vi "9401_Update Lines.vi"(8 "error in":errorcluster, 9 "DIO7:4":u32(ring) items=["Input", "Output"], 10 "DIO3:0":u32(ring) items=["Input", "Output"], 11 "Node Ptr in":T1 format="%.0x") -> (0 "error out":errorcluster, 3 "Node Ptr out":T1 format="%.0x")   [LabVIEW 2019, in "Modules.lvlib" / "9401.lvclass"]
uses:
  9401.lvclass
  <vilib>/NI VeriStand/Custom Device API/Custom Device Item Ref.ctl
  C:/Users/nitest/Desktop/Git 2019/niveristand-scan-engine-module-libraries/Source/RSI Module/RSI Module.lvclass
  <vilib>/NI VeriStand/Custom Device API/Custom Device Channel Type.ctl
  9401.lvclass/9401.ctl
  RSI Module/Channel GUIDs.vi
  RSI Module/RSI Module.lvclass
  <vilib>/NI VeriStand/Custom Device API/Custom Device API.lvlib
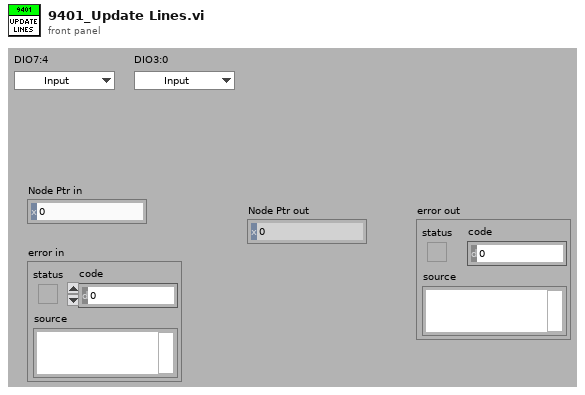
[diagram p1: front panel]
types:
  T1 = typedef "Custom Device API.lvlib/Custom Device Item Ref.ctl" = u64
  T2 = typedef "Custom Device API.lvlib/Custom Device Channel Type.ctl" = enum16{"Input", "Output"}
  T3 = typedef "Modules.lvlib/RSI Module.lvclass/Channels.ctl" = cluster{"# Input Channels":i32, "# Output Channels":i32, "Channel Type":T4, "Units":string}
  T4 = typedef "Modules.lvlib/RSI Module.lvclass/Channel Type.ctl" = enum16{"Analog", "Digital"}
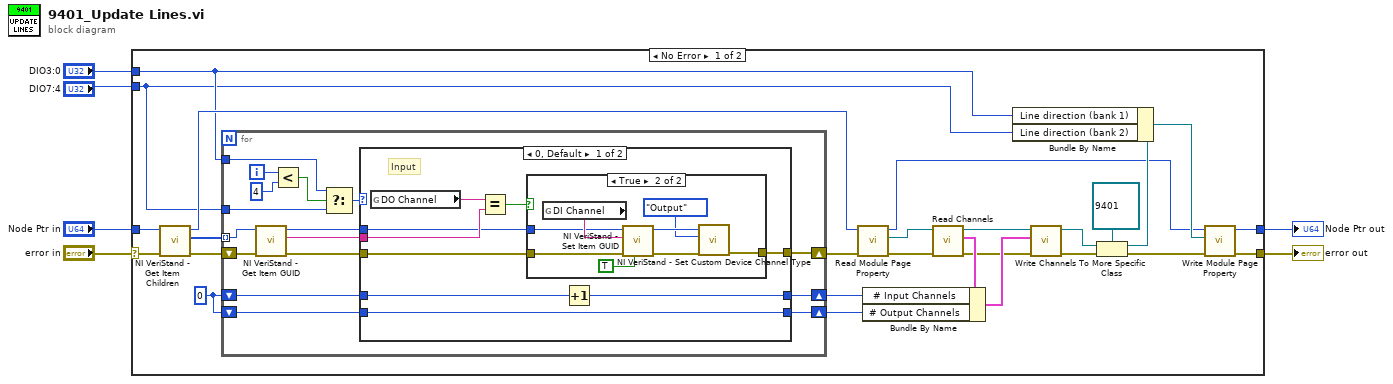
[diagram p0: block diagram]
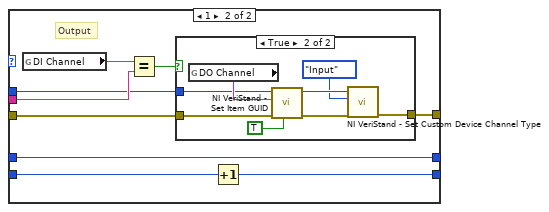
[diagram p3: hidden frame]
diagram:
  n1 = case shown="No Error" "error in" {
    selector: "error in" -> [w25 w86]
    tunnel: [w30 w86] -> w6
    tunnel: "Node Ptr in" -> [w24 w85]
    tunnel: [w26 w85] -> w4
    tunnel: "DIO3:0" -> [w20 _]
    tunnel: "DIO7:4" -> [w19 _]
    frame No Error {
      w18 = 0 ("# Input Channels")
      n2 = call <vilib>:"NI VeriStand - Get Item Children.vi"("error in (no error)"=w25, "Item Ref in"=w24) -> ("error out"=w22:errorcluster, "Child Refs"=w23:T1[], "Item Ref out"=w21:T1)  [unwired: 6 in, 1 out]
      n3 = for {
        tunnel: w23 -> [w47] mode=indexing
        shift-right: [w33] -> w17
        shift-left: w22 -> [w48]
        tunnel: w20 -> [w44]
        tunnel: w19 -> [w43]
        shift-right: [w35] -> w8
        shift-left: w18 -> [w37]
        shift-right: [w34] -> w7
        shift-left: w18 -> [w36]
        i -> [w46]
        n4 = call <vilib>:"NI VeriStand - Get Item GUID.vi"("error in (no error)"=w48, "Item Ref in"=w47) -> ("error out"=w38:errorcluster, "GUID"=w40:string, "Item Ref out"=w39:T1)  [unwired: 7 in]
        n5 = Less?(x=w46, y=4) -> (x < y?=w42:bool)
        n6 = Select(t=w44, s=w42, f=w43) -> (s? t:f=w41:u32)
        n7 = case shown="0, Default" w41 {
          tunnel: w40 -> [w56 w74]
          tunnel: w39 -> [w53 w71]
          tunnel: w38 -> [w54 w72]
          tunnel: [w52 w70] -> w33
          tunnel: w37 -> [w51 w67]
          tunnel: w36 -> [w49 w69]
          tunnel: [w50 w67] -> w35
          tunnel: [w49 w68] -> w34
          frame 0, Default {
            # "Input"
            n8 = global read "Channel GUIDs.vi" "DO Channel"() -> (w57:string)
            n9 = Equal?(x=w57, y=w56) -> (x = y?=w55:bool)
            n10 = case shown="True" w55 {
              tunnel: w54 -> [w58 w66]
              tunnel: w53 -> [_ w64]
              tunnel: [w58 w61] -> w52
              frame False {
              }
              frame True {
                n11 = global read "Channel GUIDs.vi" "DI Channel"() -> (w65:string)
                n12 = call <vilib>:"NI VeriStand - Set Item GUID.vi"("Refresh System Explorer Tree? (F)"=TRUE, "error in (no error)"=w66, "GUID"=w65, "Item Ref in"=w64) -> ("error out"=w62:errorcluster, "Item Ref out"=w63:T1)  [unwired: 6 in]
                n13 = call <vilib>:"NI VeriStand - Set Custom Device Channel Type.vi"("error in (no error)"=w62, "Type"=Custom_Device_Channel_Type."Output", "Channel Ref in"=w63) -> ("error out"=w61:errorcluster)  [unwired: 7 in, 1 out]
              }
            }
            n14 = Increment(x=w51) -> (x+1=w50:i32)
          }
          frame 1 {
            # "Output"
            n15 = global read "Channel GUIDs.vi" "DI Channel"() -> (w75:string)
            n16 = Equal?(x=w75, y=w74) -> (x = y?=w73:bool)
            n17 = case shown="True" w73 {
              tunnel: w72 -> [w76 w84]
              tunnel: w71 -> [_ w82]
              tunnel: [w76 w79] -> w70
              frame False {
              }
              frame True {
                n18 = global read "Channel GUIDs.vi" "DO Channel"() -> (w83:string)
                n19 = call <vilib>:"NI VeriStand - Set Item GUID.vi"("Refresh System Explorer Tree? (F)"=TRUE, "error in (no error)"=w84, "GUID"=w83, "Item Ref in"=w82) -> ("error out"=w80:errorcluster, "Item Ref out"=w81:T1)  [unwired: 6 in]
                n20 = call <vilib>:"NI VeriStand - Set Custom Device Channel Type.vi"("error in (no error)"=w80, "Type"=Custom_Device_Channel_Type."Input", "Channel Ref in"=w81) -> ("error out"=w79:errorcluster)  [unwired: 7 in, 1 out]
              }
            }
            n21 = Increment(x=w69) -> (x+1=w68:i32)
          }
        }
      }
      n22 = call "Read Module Page Property.vi"("error in (no error)"=w17, "Node Ptr In"=w21) -> ("error out"=w11:errorcluster, "RSI Module"=w12:refnum<class "RSI Module.lvclass">, "Node Ptr Out"=w29:T1)  [unwired: 7 in]
      n23 = call "Read Channels.vi"("error in (no error)"=w11, "RSI Module in"=w12) -> ("error out"=w13:errorcluster, "Channels"=w15:T3, "RSI Module out"=w14:refnum<class "RSI Module.lvclass">)  [unwired: 7 in]
      n24 = Bundle By Name(cluster=w15, "# Input Channels"=w8, "# Output Channels"=w7) -> (w16:T3)
      n25 = call "Write Channels.vi"("error in (no error)"=w13, "Channels"=w16, "RSI Module in"=w14) -> ("error out"=w9:errorcluster, "RSI Module out"=w10:refnum<class "RSI Module.lvclass">)  [unwired: 7 in]
      n26 = To More Specific Class(target class=refnum<class "9401.lvclass"> refnum ("9205 in"), reference=w10, error in=w9) -> (specific class reference=w31:refnum<class "9401.lvclass">, error out=w28:errorcluster)
      n27 = Bundle By Name(cluster=w31, "Line direction (bank 1)"=w20, "Line direction (bank 2)"=w19) -> (w32:refnum<class "9401.lvclass">)
      n28 = call "Write Module Page Property.vi"("error in (no error)"=w28, "RSI Module"=w32, "Node Ptr In"=w29) -> ("error out"=w30:errorcluster, "Node Ptr Out"=w26:T1)  [unwired: 6 in, 1 out]
    }
    frame Error {
    }
  }
  "error out" <- w6
  "Node Ptr out" <- w4
